vi "PwmOut.vi"(8 "error in (no error)":errorcluster, 9 "Existing Obj Name":string, 10 "Pin":string, 11 "mbed_LVLibrary.lvlib:mbed.lvclass":refnum<class "mbed.lvclass">) -> (0 "error out":errorcluster, 1 "Assigned Name":string, 3 "PwmOut.lvclass 2":refnum<class "PwmOut.lvclass">)   [LabVIEW 2011, in "mbed_LVLibrary.lvlib" / "PwmOut.lvclass"]
uses:
  PwmOut.lvclass
  Transport Mechanisms/mbed/mbed.lvclass
  PwmOut.lvclass/PwmOut.ctl
  <vilib>/regexp/Match Regular Expression.xnode
panel:
  in  "PwmOut.lvclass":refnum<class "PwmOut.lvclass">
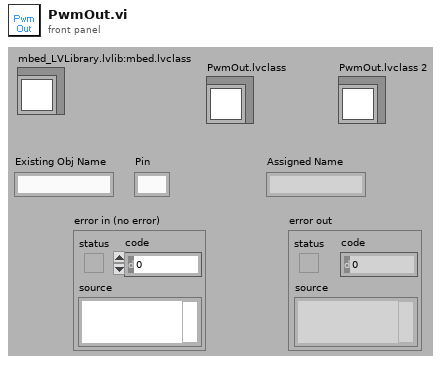
[diagram p1: front panel]
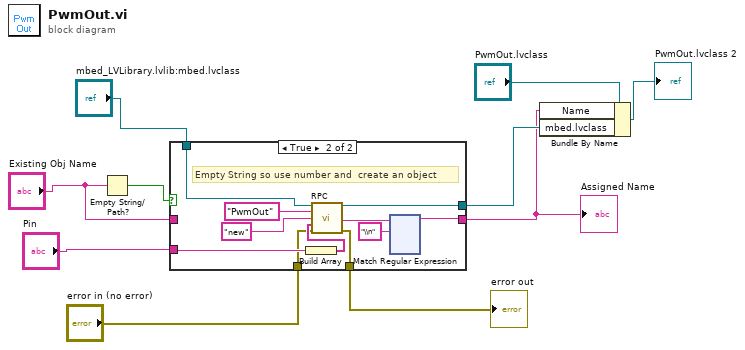
[diagram p0: block diagram]
diagram:
  n1 = Empty String/Path?(string/path="Existing Obj Name") -> (empty?=w7:bool)
  n2 = case shown="True" w7 {
    tunnel: "Existing Obj Name" -> [w13 _]
    tunnel: [w13 w20] -> w8
    tunnel: "mbed_LVLibrary.lvlib:mbed.lvclass" -> [w12 w24]
    tunnel: [w12 w21] -> w9
    tunnel: "Pin" -> [_ w16]
    tunnel: "error in (no error)" -> [w11 w15]
    tunnel: [w11 w14] -> w2
    frame False {
      # "String present so just set the class name"
    }
    frame True {
      # "Empty String so use number and  create an object"
      n3 = Build Array(w16) -> (w17:string[])
      n4 = call-dynamic "RPC.vi"("mbed in"=w24, "Name"="PwmOut", "method"="new", "Args"=w17, "error in (no error)"=w15) -> ("mbed out"=w21:refnum<class "mbed.lvclass">, "RPC Result"=w19:string, "error out"=w14:errorcluster)  [unwired: 8 in]
      n5 = xnode "Match Regular Expression"("input string"=w19, "regular expression"="\\n") -> ("before match"=w20:string)  [unwired: 4 in, 4 out]
    }
  }
  "Assigned Name" <- w8
  "error out" <- w2
  n6 = Bundle By Name(cluster="PwmOut.lvclass", "Name"=w8, "mbed.lvclass"=w9) -> (→"PwmOut.lvclass 2":refnum<class "PwmOut.lvclass">)
